vi "Data Read.vi"(7 "Retry Attempts (0)":i32 min=0, 8 "error in (no error)":errorcluster, 10 "Bytes to read":u32, 11 "VISA Refnum in":refnum<visa-resource-name>) -> (0 "error out":errorcluster, 2 "read buffer":string, 3 "VISA Refnum out":refnum<visa-resource-name>)   [LabVIEW 2020, in "driver_chromtech_nextgen_pump.lvlib"]
uses:
  driver_chromtech_nextgen_pump.lvlib
  <vilib>/Utility/sysdir.llb/System Directory Type.ctl
panel:
  out "Retries":i32
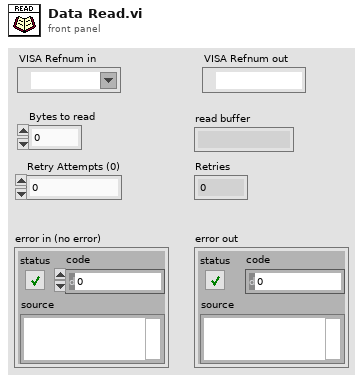
[diagram p1: front panel]
types:
  T1 = typedef "System Directory Type.ctl" = i32
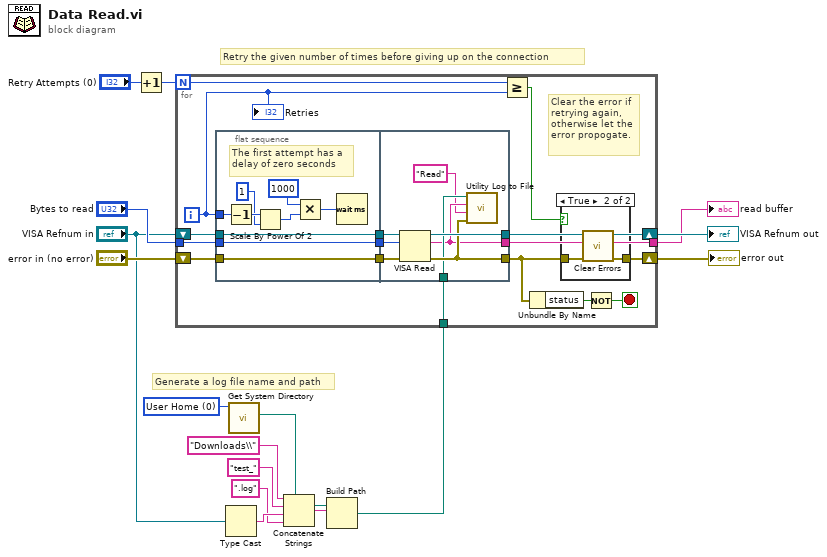
[diagram p0: block diagram]
diagram:
  w7 = T1 0 items=["User Home"=0, "User Desktop"=1, "User Documents"=2, "User Application Data"=3, "User Preferences"=4, "User Temporary"=5, "Public Documents"=6, "Public Application Data"=7, "Public Preferences"=8, "Public Cache"=13, "System Core Libraries"=9, "System Installed Libraries"=10, "Application Files"=11, "Boot Volume Root"=12] ("system directory type")
  # "Retry the given number of times before giving up on the connection"
  # "Generate a log file name and path"
  n1 = Increment(x="Retry Attempts (0)") -> (x+1=w1:i32)
  n2 = Type Cast(x="VISA Refnum in") -> (*(type *) &x=w11:string)  [unwired: 1 in]
  n3 = call <vilib>:"Get System Directory.vi"("system directory type"=w7) -> ("system directory"=w8:path)  [unwired: 10 in]
  n4 = Concatenate Strings("Downloads\\", "test_", w11, ".log") -> (w10:string)
  n5 = Build Path(base path=w8, name or relative path=w10) -> (appended path=w3:path)
  n6 = for {
    N: w1 -> [w17]
    tunnel: "Bytes to read" -> [w31]
    tunnel: [w27] -> w13
    tunnel: w3 -> [w28]
    shift-right: [w20] -> w4
    shift-left: "error in (no error)" -> [w30]
    shift-right: [w32] -> w16
    shift-left: "VISA Refnum in" -> [w29]
    i -> [w18]
    stop <- w21 stop-if-true
    # "Clear the error if\nretrying again,\notherwise let the\nerror propogate."
    n7 = flat-sequence {
      tunnel: w29 -> [w42]
      tunnel: w30 -> [w43]
      tunnel: w31 -> [w44]
      tunnel: [w44] -> w26
      tunnel: [w43] -> w25
      tunnel: [w42] -> w24
      tunnel: w18 -> [w36]
      tunnel: [w52] -> w32
      tunnel: [w48] -> w23
      tunnel: w28 -> [w47]
      tunnel: [w46] -> w27
      tunnel: w26 -> [w51]
      tunnel: w25 -> [w50]
      tunnel: w24 -> [w49]
      frame #0 {
        # "The first attempt has a \ndelay of zero seconds"
        n8 = Decrement(x=w36) -> (x-1=w38:i32)
        n9 = Scale By Power Of 2(n=w38, x=1) -> (x*2^n=w41:i32)
        n10 = Multiply(x=1000, y=w41) -> (x*y=w39:i32)
        n11 = Wait (ms)(milliseconds to wait=w39) -> ()  [unwired: 1 out]
      }
      frame #1 {
        n12 = VISA Read(VISA resource name=w49, byte count=w51, error in (no error)=w50) -> (VISA resource name out=w52:refnum<visa-resource-name>, read buffer=w46:string, error out=w48:errorcluster)  [unwired: 1 out]
        n13 = call "Utility Log to File.vi"("error in (no error)"=w48, "Additional Notes"="Read", "Command"=w46, "Log File Path"=w47) -> ()  [unwired: 7 in, 1 out]
      }
    }
    n14 = Greater Or Equal?(x=w17, y=w18) -> (x >= y?=w19:bool)
    n15 = Unbundle By Name(w23) -> ("status"=w22:bool)
    n16 = case shown="True" w19 {
      tunnel: w23 -> [w33 w35]
      tunnel: [w33 w34] -> w20
      frame False {
      }
      frame True {
        n17 = call <vilib>:"Clear Errors.vi"("error in (no error)"=w35) -> ("error out"=w34:errorcluster)  [unwired: 5 in, 1 out]
      }
    }
    n18 = Not(x=w22) -> (.not. x?=w21:bool)
    "Retries" <- w18
  }
  "read buffer" <- w13
  "VISA Refnum out" <- w16
  "error out" <- w4
